vi "power vs time PID - V1.vi"(6 "delta time(sec)":dbl=300.0, 7 "control set temperature PID?":bool, 10 "sweep folder path":path) -> (0 "next set temperature":dbl, 1 "set temperature points":dbl[](array[numeric]), 2 "time points (min)":dbl[](array[numeric]))   [LabVIEW 2012]
uses:
  next chunk read-write PID -- action.ctl
  ctl -- name dispatcher -- action.ctl
  file -- 9w path.vi
  array -- find index - real.vi
  array -- interpolate -- i.vi
  ctl -- name dispatcher.vi
  Q -- check range -- i -- real.vi
  Q - not nan -- real.vi
  <vilib>/Utility/libraryn.llb/Check if File or Folder Exists.vi
  file -- read list of lines.vi
  parse -- find first line.vi
  parse -- get list of matches -- numbers.vi
  <vilib>/Utility/file.llb/Write To Spreadsheet File.vi
  <vilib>/Utility/file.llb/Write To Spreadsheet File (string).vi
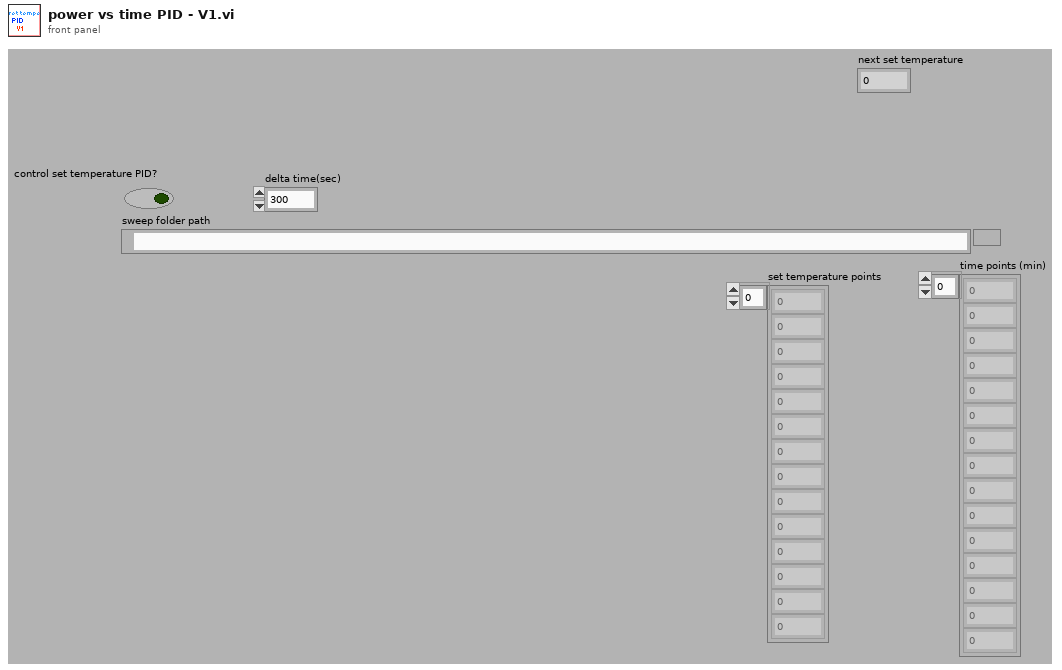
[diagram p1: front panel]
types:
  T1 = typedef "ctl -- name dispatcher -- action.ctl" = enum16{"peak frequency", "peak frequency DUMP", "peak gamma DUMP", "peak gamma", "peak frequency TEST", "peak gamma TEST", "ultrasonic power", "time in gamma", "set temperature ", "set temperature timer", "peak default gamma", "last scan file", "peak freq gamma TEST", "peak NAMES", "errors", "P_I_D", "P", "I", "D", "power vs time"}
  T2 = typedef "next chunk read-write PID -- action.ctl" = enum16{"read", "interpolate", "append col", "write", "write PID col", "append PID col", "interpolate - bezier"}
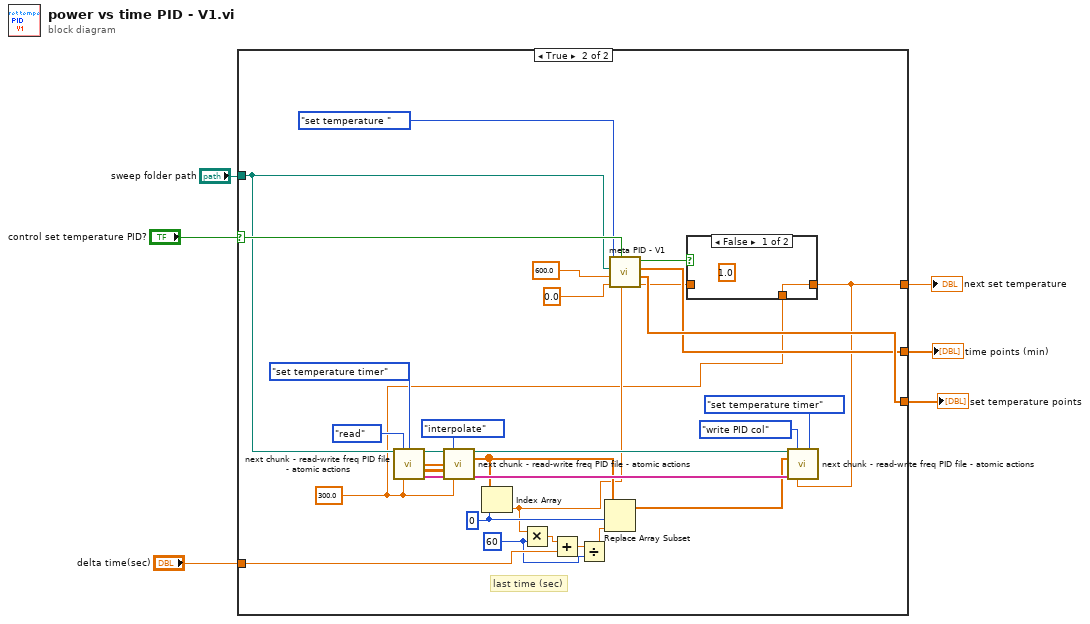
[diagram p0: block diagram]
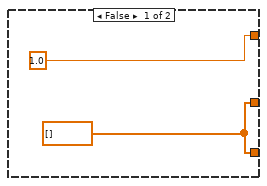
[diagram p2: hidden frame]
diagram:
  n1 = case shown="True" "control set temperature PID?" {
    selector: "control set temperature PID?" -> [_ w36]
    tunnel: "sweep folder path" -> [_ w30]
    tunnel: "delta time(sec)" -> [_ w22]
    tunnel: [1.0 ("upper") w10] -> w3
    tunnel: [w7 w34] -> w2
    tunnel: [w7 w35] -> w1
    frame False {
      w7 = dbl[] [] ("temperatures")
    }
    frame True {
      w11 = 300.0 ("temperature")
      w20 = 0 ("index")
      w15 = 60
      # "last time (sec)"
      n2 = call "next chunk - read-write freq PID file - atomic actions .vi"("sweep folder path"=w30, "PID action"=next_chunk_read-write_PID_--_action."read", "ctl kind IN"=ctl_--_name_dispatcher_--_action."set temperature timer", "temperature"=w11) -> ("sweep folder path out"=w29:path, "temperatures"=w25:dbl[], "frequencies"=w24:dbl[][], "header"=w26:string[])  [unwired: 7 in, 1 out]
      n3 = call "next chunk - read-write freq PID file - atomic actions .vi"("PID action"=next_chunk_read-write_PID_--_action."interpolate", "temperatures IN"=w25, "frequencies IN"=w24, "header IN"=w26, "temperature"=w11) -> ("PID freq"=w16:dbl[], "header"=w21:string[])  [unwired: 6 in, 3 out]
      n4 = Index Array(array=w16, index=w20) -> (element=w13:dbl)
      n5 = Multiply(x=w13, y=w15) -> (x*y=w14:dbl)
      n6 = Add(x=w14, y=w22) -> (x+y=w18:dbl)
      n7 = Divide(x=w18, y=w15) -> (x/y=w17:dbl)
      n8 = Replace Array Subset(array=w16, new element=w17, index=w20) -> (w19:dbl[])
      n9 = call "meta PID - V1.vi"("input parameter"=w13, "control?"=w36, "lower limit"=0.0 ("lower"), "upper limit"=600.0 ("upper"), "sweep folder path"=w30, "ctl name dispatch"=ctl_--_name_dispatcher_--_action."set temperature ") -> ("bezier output"=w12:dbl, "frequencies"=w35:dbl[], "temperatures"=w34:dbl[], "ok"=w33:bool)  [unwired: 2 in]
      n10 = case shown="False" w33 {
        tunnel: [w39 w40] -> w10
        tunnel: w12 -> [_ w40]
        tunnel: w11 -> [w39 _]
        frame False {
          (unwired) 1.0 ("upper")
        }
        frame True {
        }
      }
      n11 = call "next chunk - read-write freq PID file - atomic actions .vi"("sweep folder path"=w29, "PID action"=next_chunk_read-write_PID_--_action."write PID col", "ctl kind OUT"=ctl_--_name_dispatcher_--_action."set temperature timer", "PID freq IN"=w19, "header IN"=w21, "temperature"=w10) -> ()  [unwired: 5 in, 5 out]
    }
  }
  "next set temperature" <- w3
  "time points (min)" <- w2
  "set temperature points" <- w1
